vi "GetBoardCorners.vi"(8 "error in (no error)":errorcluster, 11 "Board in":refnum<class "Board.lvclass">) -> (0 "error out":errorcluster, 2 "BoardCorners":T1, 3 "Board out":refnum<class "Board.lvclass">)   [LabVIEW 2015, in "TronviewGame.lvlib" / "Board.lvclass"]
uses:
  Board.lvclass
  BoardCorners.ctl
  Position.ctl
  Board.lvclass/Board.ctl
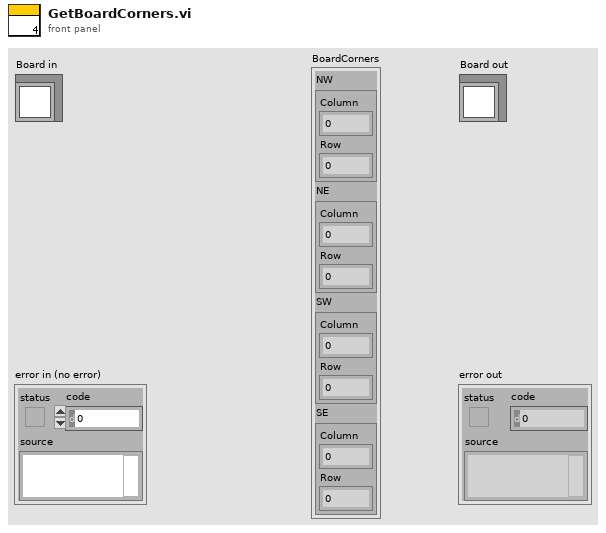
[diagram p1: front panel]
types:
  T1 = typedef "TronviewGame.lvlib/Board.lvclass/BoardCorners.ctl" = cluster{"NW":T2, "NE":T2, "SW":T2, "SE":T2}
  T2 = typedef "TronviewGame.lvlib/Board.lvclass/Position.ctl" = cluster{"Column":i32, "Row":i32}
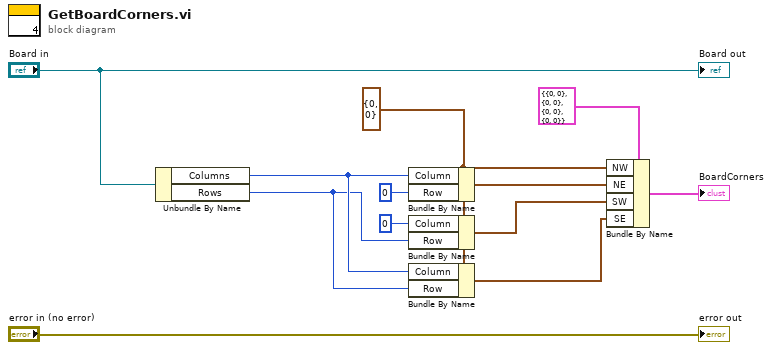
[diagram p0: block diagram]
diagram:
  w8 = T2 {"Column"=0, "Row"=0} ("Position")
  n1 = Unbundle By Name("Board in") -> ("Columns"=w5:u32, "Rows"=w4:u32)
  n2 = Bundle By Name(cluster=w8, "Column"=w5, "Row"=u32 0) -> (w7:T2)
  n3 = Bundle By Name(cluster=w8, "Column"=u32 0, "Row"=w4) -> (w3:T2)
  n4 = Bundle By Name(cluster=w8, "Column"=w5, "Row"=w4) -> (w2:T2)
  n5 = Bundle By Name(cluster=T1 {"NW"={"Column"=0, "Row"=0}, "NE"={"Column"=0, "Row"=0}, "SW"={"Column"=0, "Row"=0}, "SE"={"Column"=0, "Row"=0}} ("Corners"), "NW"=w8, "NE"=w7, "SW"=w3, "SE"=w2) -> (→"BoardCorners":T1)
  "error out" <- "error in (no error)"
  "Board out" <- "Board in"
